vi "createRegisters.vi"() -> (2 "modRegisters":T1={"numberOfInterleaves"="Register", "Enable"="Register", "triangleInc"="Register", "Deadband"="Register", "Enabled"="Register"}, 3 "settingsReg":T2={"numberOfInterleaves"="", "rampRate"="", "manualInput"="", "perturbAmp"="", "perturbAngleInc"="", "reset"="", "state"="", "gains"="", "Currents"="Currents"})   [LabVIEW 2017, in "BuckBoost.lvlib"]
uses:
  BuckBoost.lvlib
  contSettings.ctl
  modRegisters.ctl
  <vilib>/rvi/eio/common/nirviEmuReportErrorAndStop.vi
  <vilib>/rvi/DataTransferAndStorage/Container/Common/niFpgaContainerSetEmuInfo.vi
  <vilib>/rvi/DataTransferAndStorage/Container/Common/niFpgaContainerGetUniqueNameForEmu.vi
  <vilib>/rvi/LocalResourceManager/LocalResourceManager.xnode
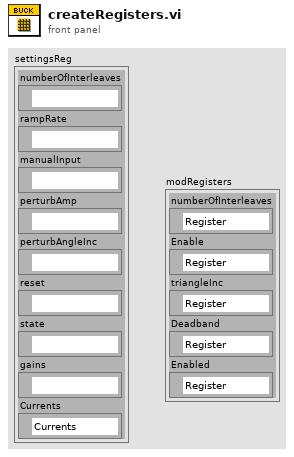
[diagram p1: front panel]
types:
  T1 = typedef "BuckBoost.lvlib/modRegisters.ctl" = cluster{"numberOfInterleaves":refnum<k21>, "Enable":refnum<k21>, "triangleInc":refnum<k21>, "Deadband":refnum<k21>, "Enabled":refnum<k21>}
  T2 = typedef "BuckBoost.lvlib/contSettings.ctl" = cluster{"numberOfInterleaves":refnum<k21>, "rampRate":refnum<k21>, "manualInput":refnum<k21>, "perturbAmp":refnum<k21>, "perturbAngleInc":refnum<k21>, "reset":refnum<k21>, "state":refnum<k21>, "gains":refnum<k21>, "Currents":refnum<k21>}
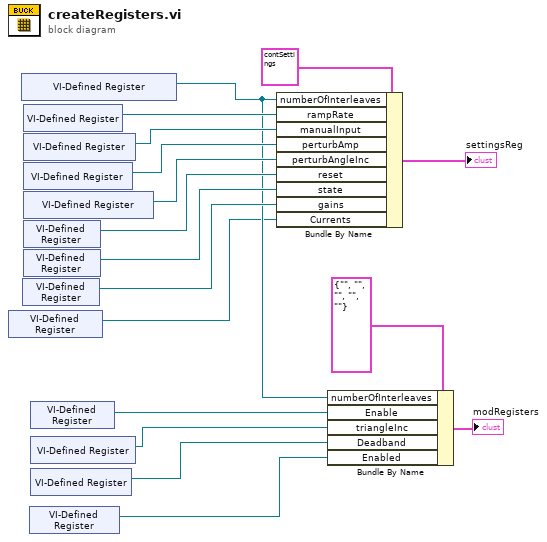
[diagram p0: block diagram]
diagram:
  n1 = xnode "VI-Defined Register"() -> ("Register Out"=w1:refnum<k21>)
  n2 = xnode "VI-Defined Register"() -> ("Register Out"=w7:refnum<k21>)
  n3 = xnode "VI-Defined Register"() -> ("Register Out"=w16:refnum<k21>)
  n4 = xnode "VI-Defined Register"() -> ("Register Out"=w10:refnum<k21>)
  n5 = xnode "VI-Defined Register"() -> ("Register Out"=w11:refnum<k21>)
  n6 = xnode "VI-Defined Register"() -> ("Register Out"=w12:refnum<k21>)
  n7 = xnode "VI-Defined Register"() -> ("Register Out"=w13:refnum<k21>)
  n8 = xnode "VI-Defined Register"() -> ("Register Out"=w14:refnum<k21>)
  n9 = xnode "VI-Defined Register"() -> ("Register Out"=w15:refnum<k21>)
  n10 = xnode "VI-Defined Register"() -> ("Register Out"=w2:refnum<k21>)
  n11 = xnode "VI-Defined Register"() -> ("Register Out"=w6:refnum<k21>)
  n12 = xnode "VI-Defined Register"() -> ("Register Out"=w5:refnum<k21>)
  n13 = xnode "VI-Defined Register"() -> ("Register Out"=w4:refnum<k21>)
  n14 = Bundle By Name(cluster=T2 {"numberOfInterleaves"="", "rampRate"="", "manualInput"="", "perturbAmp"="", "perturbAngleInc"="", "reset"="", "state"="", "gains"="", "Currents"="Currents"} ("settings"), "numberOfInterleaves"=w7, "rampRate"=w10, "manualInput"=w11, "perturbAmp"=w12, "perturbAngleInc"=w13, "reset"=w14, "state"=w15, "gains"=w16, "Currents"=w1) -> (→"settingsReg":T2)
  n15 = Bundle By Name(cluster=T1 {"numberOfInterleaves"="", "Enable"="", "triangleInc"="", "Deadband"="", "Enabled"=""} ("modRegisters"), "numberOfInterleaves"=w7, "Enable"=w6, "triangleInc"=w5, "Deadband"=w4, "Enabled"=w2) -> (→"modRegisters":T1)
